vi "WriteStoreDataIngoHeucke.vi"(1 "Spots":T1[](array[typedef]) {"F2-Value overall" format="%.2f"; "tauerror" format="%.2f"; "Lifetime[ns]" format="%.2f"; "F2-Value TAC" format="%.2f"}, 2 "Enum":enum16{"Save", "Control"}(ring), 3 "Image Path":refnum<vi>) -> (0 "already x spots":i16)   [LabVIEW 2009]
uses:
  spotproperties.ctl
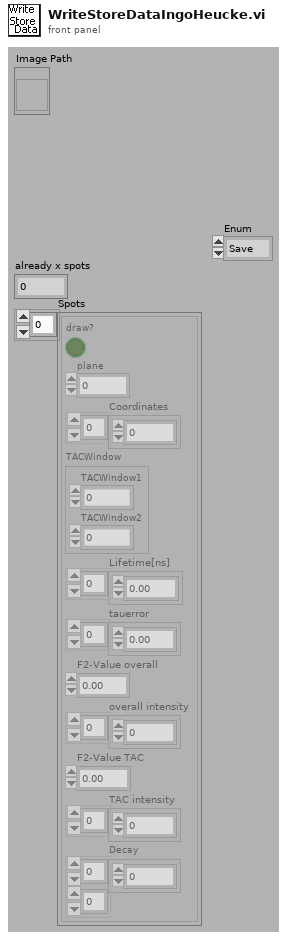
[diagram p1: front panel]
types:
  T1 = typedef "spotproperties.ctl" = cluster{"draw?":bool, "plane":u32, "Coordinates":i32[], "TACWindow":cluster{"TACWindow1":i32, "TACWindow2":i32}, "Lifetime[ns]":ext[], "tauerror":dbl[], "F2-Value overall":dbl, "overall intensity":u32[], "F2-Value TAC":dbl, "TAC intensity":u32[], "Decay":u32[][]}
  T2 = enum16{"Display", "change", "Get", "Set", "Set Ken"}
  T3 = enum16{"open", "open or create", "create or replace", "create", "open (read only)"}
  T4 = enum16{"read/write", "read-only", "write-only", "write-only (truncate)"}
  T5 = typedef "Settings.ctl" = cluster{"threshold":cluster{"max":u32, "min":u32}, "RGB or false color":bool, "16bit":bool, "log/lin axis":u16, "spotsize button":bool, "Pixelsize":u16, "autoscale x":bool, "autoscale y":bool, "correlation":bool, "ADC-Resolution":i32, "F2-lifetime":cluster{"display tau":bool, "display F2":bool, "Palette Number lifetime":enum32{"Gray", "Binary", "Gradient", "Rainbow", "Temperature"}, "Palette Number F2":enum32{"Gray", "Binary", "Gradient", "Rainbow", "Temperature"}, "max tau-Value":dbl, "min tau-Value":dbl, "max F2-Value":dbl, "min F2-Value":dbl}, "TAC-Window 1":u16, "TAC-Window 2":u16, "false color palette":cluster{"1":u32, "2":u32, "3":u32, "4":u32, "5":u32, "6":u32, "7":u32, "8":u32, "8 2":u32, "8 3":u32, "8 4":u32, "8 5":u32}}
  T6 = typedef "FIFOSettings_BH.ctt" = cluster{"Measurement":cluster{"Binning (ms)":sgl, "External Trigger Condition":u16, "Stop Condition:":u16, "Stop Count":dbl, "Buffer Size (Photons)":u16, "No of Channels":u16, "Ext Latch Delay":i16}, "ADC":cluster{"Module":u16, "ADC Resolution":i32, "Dither Range":i16, "Count Increment":i16, "Macro Time Clock":i16}, "SYNC":cluster{"SYNC ZC Level (mV)":sgl, "SYNC Freq Divider":i16, "SYNC Holdoff (ns)":sgl, "SYNC Threshold (mV)":sgl}, "TAC":cluster{"TAC Range (ns)":sgl, "TAC Gain":i16, "TAC Offset (%)":sgl, "TAC Limit Low (%)":sgl, "TAC Limit High (%)":sgl}, "CFD":cluster{"CFD Limit Low (mV)":sgl, "CFD Limit High (mV)":sgl, "CFD ZC Level (mV)":sgl, "CFD Holdoff (ns)":sgl}}
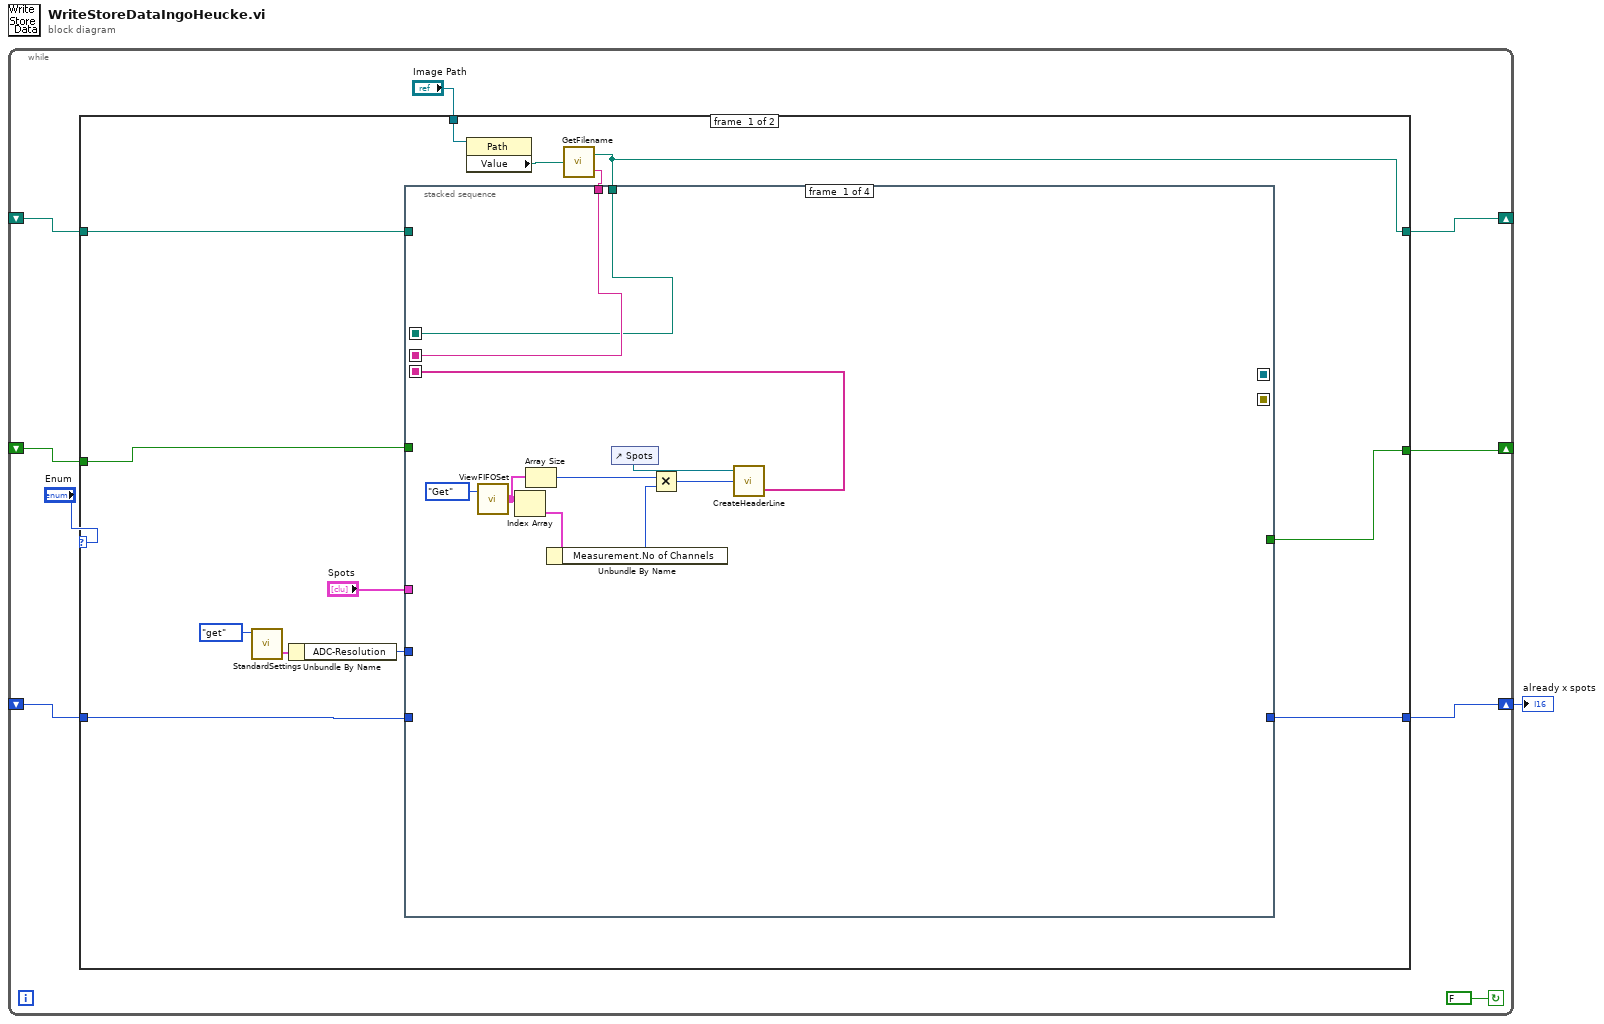
[diagram p0: block diagram]
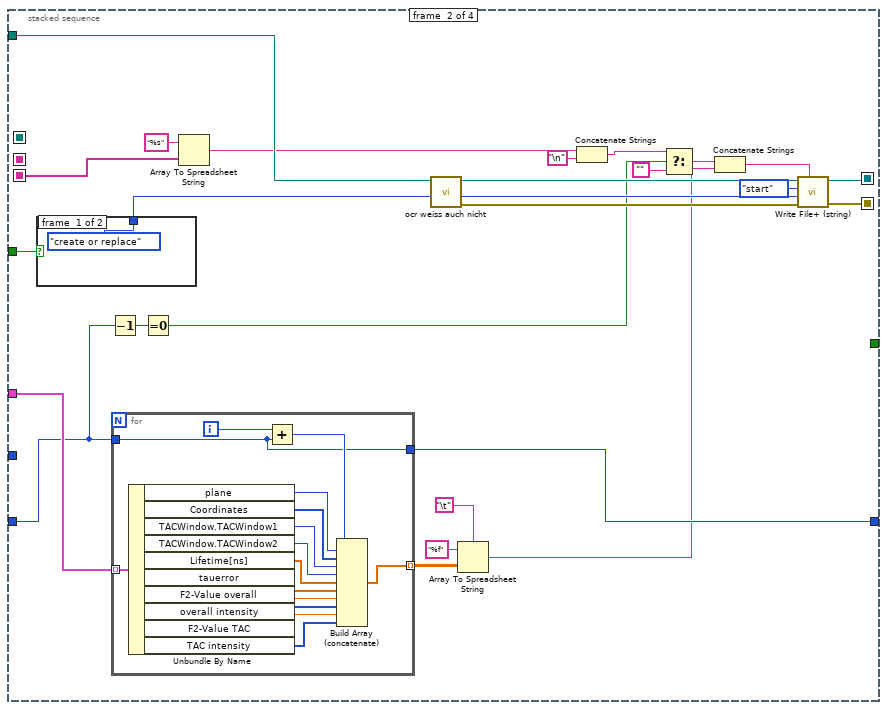
[diagram p2: hidden frame]
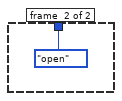
[diagram p3: hidden frame]
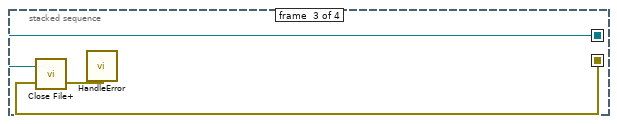
[diagram p4: hidden frame]
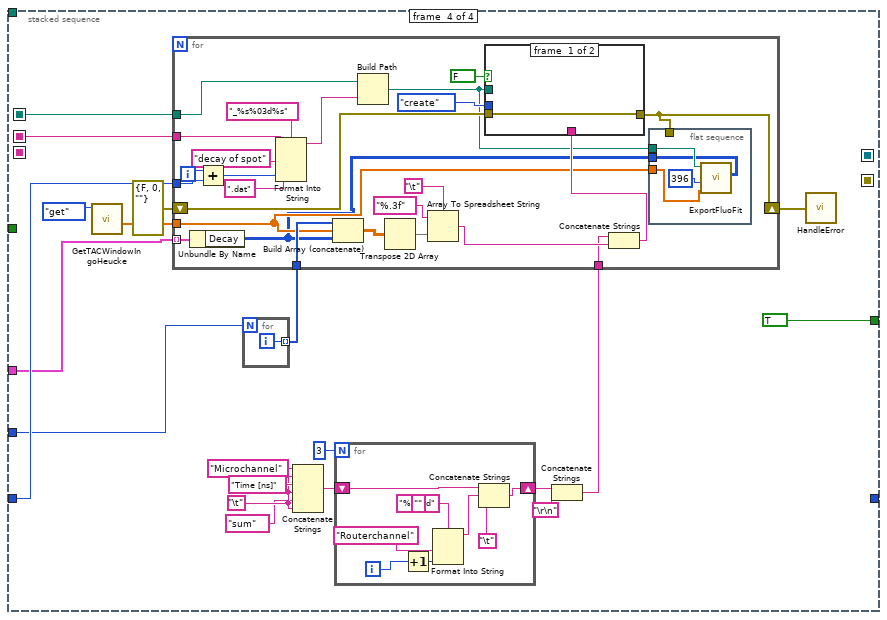
[diagram p5: hidden frame]
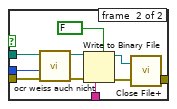
[diagram p6: hidden frame]
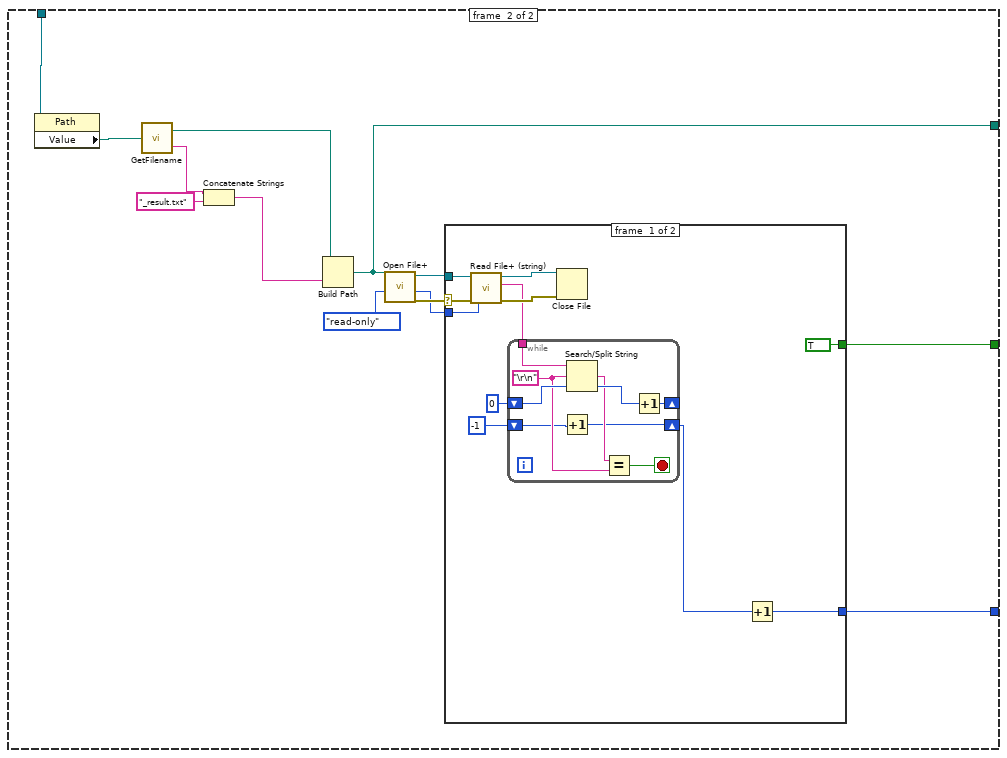
[diagram p7: hidden frame]
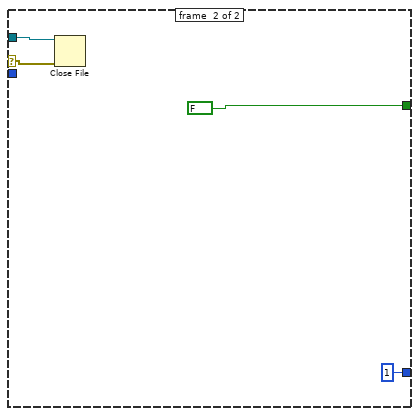
[diagram p8: hidden frame]
diagram:
  n1 = while {
    shift-right: [w8] -> _
    shift-left: _ -> [w7]
    shift-right: [w6] -> w1
    shift-left: _ -> [w5]
    shift-right: [w4] -> _
    shift-left: _ -> [w3]
    stop <- FALSE continue-if-true
    n2 = case shown="\"Save\", Default" "Enum" {
      tunnel: [w23 w161] -> w8
      tunnel: w7 -> [w22 _]
      tunnel: [w21 w149] -> w6
      tunnel: w5 -> [w15 _]
      tunnel: [w11 w151] -> w4
      tunnel: w3 -> [w20 _]
      tunnel: "Image Path" -> [w13 w150]
      frame #0 {
        n3 = call "StandardSettings.vi"("Enum"=enum16{"Load", "get", "Save", "set"}."get") -> ("StandardSettings"=w18:T5)  [unwired: 4 in]
        n4 = Unbundle By Name(w18) -> ("ADC-Resolution"=w17:i32)
        n5 = property class="Path"(reference=w13) -> ("Value"=w14:path)  [unwired: 1 in, 2 out]
        n6 = call "GetFilename.vi"("Value"=w14) -> ("base path"=w11:path, "name"=w12:string)
        n7 = stacked-sequence {
          seq-local: [w24 _ _ _] -> [_ _ _ w99]
          seq-local: [w25 _ _ _] -> [_ _ _ w87]
          seq-local: [w32 _ _ _] -> [_ w45 _ _]
          seq-local: [_ w58 _ _] -> [_ _ w79 _]
          seq-local: [_ w57 _ _] -> [_ _ w78 _]
          tunnel: "Spots" -> [_ w56 _ w84]
          tunnel: [_ _ _ TRUE] -> w23
          tunnel: w22 -> [_ w49 _ _]
          tunnel: [_ w48 _ _] -> w21
          tunnel: w15 -> [_ w41 _ w91]
          tunnel: w20 -> [_ w46 _ _]
          tunnel: w17 -> [_ _ _ w83]
          tunnel: w12 -> [w25 _ _ _]
          tunnel: w11 -> [w24 _ _ _]
          frame #0 {
            n8 = call "ViewFIFOSet.vi"("Enum"=T2."Get") -> ("FIFO Settings (Array)"=w27:T6[])  [unwired: 1 in]
            n9 = Index Array(array=w27) -> (element=w30:T6)  [unwired: 1 in]
            n10 = Array Size(array=w27) -> (size(s)=w28:i32)
            n11 = Unbundle By Name(w30) -> ("Measurement.No of Channels"=w29:u16)
            n12 = control-ref of="Spots"() -> (w33:refnum<vi>)
            n13 = Multiply(x=w28, y=w29) -> (x*y=w26:i32)
            n14 = call "CreateHeaderLine.vi"("No of channels"=w26, "Spots 3"=w33) -> ("Headline array"=w32:string[])  [unwired: 2 in]
          }
          frame #1 {
            n15 = case shown="True" w49 {
              tunnel: [T3."create or replace" ("function (open:0)") T3."open" ("function (open:0)")] -> w59
              frame #0 {
              }
              frame #1 {
              }
            }
            n16 = Decrement(x=w41) -> (x-1=w42:i16)
            n17 = for {
              tunnel: w56 -> [w76] mode=indexing
              tunnel: [w75] -> w55 mode=indexing
              tunnel: [w72] -> w48
              tunnel: w41 -> [w72]
              i -> [w74]
              n18 = Unbundle By Name(w76) -> ("plane"=w71:u32, "Coordinates"=w70:i32[], "TACWindow.TACWindow1"=w69:i32, "TACWindow.TACWindow2"=w68:i32, "Lifetime[ns]"=w67:ext[], "tauerror"=w66:dbl[], "F2-Value overall"=w65:dbl, "overall intensity"=w64:u32[], "F2-Value TAC"=w63:dbl, "TAC intensity"=w62:u32[])
              n19 = Add(x=w74, y=w72) -> (x+y=w73:i32)
              n20 = Build Array (concatenate)(w73, w71, w70, w69, w68, w67, w66, w65, w64, w63, w62) -> (w75:ext[])
            }
            n21 = Equal To 0?(x=w42) -> (x = 0?=w40:bool)
            n22 = Array To Spreadsheet String(array=w45, 3:"%s" ("format string")) -> (spreadsheet string=w43:string)  [unwired: 1 in]
            n23 = call "ocr weiss auch nicht.vi"("function (open:0)"=w59, "file path"=w46) -> ("error out"=w52:errorcluster, "file size (bytes)"=w50:i32, "refnum"=w53:refnum<file>)  [unwired: 6 in, 1 out]
            n24 = Array To Spreadsheet String(delimiter (Tab)="\t", array=w55, 3:"%f" ("format string")) -> (spreadsheet string=w36:string)
            n25 = Concatenate Strings(w43, "\n") -> (w39:string)
            n26 = Select(t=w39, s=w40, f="") -> (s? t:f=w37:string)
            n27 = Concatenate Strings(w37, w36) -> (w35:string)
            n28 = call "Write File+ (string).vi"("string"=w35, "error in (no error)"=w52, "pos offset (bytes:0)"=w50, "pos mode (rel. to end:1)"=enum16{"start", "end", "current"}."start", "refnum"=w53) -> ("error out"=w57:errorcluster, "dup refnum"=w58:refnum<file>)  [unwired: 2 in, 1 out]
          }
          frame #2 {
            n29 = call "Close File+.vi"("error in (no error)"=w78, "refnum"=w79) -> ("error out"=w77:errorcluster)  [unwired: 3 in, 2 out]
            n30 = call "HandleError.vi"("error in (no error)"=w77) -> ()
          }
          frame #3 {
            w86 = "\t"
            n31 = call "GetTACWindowIngoHeucke.vi"("Enum"=enum16{"ini", "get", "quick"}."get") -> ("x-values"=w80:dbl[])  [unwired: 1 in, 8 out]
            n32 = for {
              N: w83 -> [_]
              tunnel: [w100] -> w89 mode=indexing
              i -> [w100]
            }
            n33 = Concatenate Strings("Microchannel" ("string"), w86, "Time [ns]" ("string"), w86, "sum" ("string"), w86) -> (w93:string)
            n34 = for {
              N: 3 -> [_]
              shift-right: [w108] -> w97
              shift-left: w93 -> [w107]
              i -> [w105]
              (unwired) "%s %d" ("format string")
              n35 = Increment(x=w105) -> (x+1=w104:i32)
              n36 = Format Into String(format string="", "Routerchannel", w104) -> (resulting string=w102:string)  [unwired: 2 in, 1 out]
              n37 = Concatenate Strings(w107, w102, "\t") -> (w108:string)
            }
            n38 = Concatenate Strings(w97, "\r\n") -> (w96:string)
            n39 = for {
              tunnel: w84 -> [w133] mode=indexing
              tunnel: w99 -> [w132]
              tunnel: w80 -> [w113]
              shift-right: [w111] -> w81
              shift-left: errorcluster {"status"=FALSE, "code"=0, "source"=""} ("error out") -> [w127]
              tunnel: w96 -> [w124]
              tunnel: w91 -> [w119]
              tunnel: w87 -> [w114]
              tunnel: w89 -> [w115]
              i -> [w120]
              n40 = Unbundle By Name(w133) -> ("Decay"=w109:u32[][])
              n41 = Add(x=w120, y=w119) -> (x+y=w118:i32)
              n42 = Format Into String(format string="_%s%03d%s", initial string=w114, "decay of spot", w118, ".dat" ("replace string (\"\")")) -> (resulting string=w122:string)  [unwired: 1 in, 1 out]
              n43 = Build Array (concatenate)(w115, w113, w109) -> (w130:dbl[][])
              n44 = Build Path(base path=w132, name or relative path=w122) -> (appended path=w112:path)
              n45 = Transpose 2D Array(2D array=w130) -> (transposed array=w129:dbl[][])
              n46 = Array To Spreadsheet String(delimiter (Tab)="\t", array=w129, 3:"%.3f" ("format string")) -> (spreadsheet string=w126:string)
              n47 = Concatenate Strings(w124, w126) -> (w125:string)
              n48 = case shown="False" FALSE {
                tunnel: w127 -> [w134 w140]
                tunnel: w125 -> [_ w139]
                tunnel: T3."create" ("function (open:0)") -> [_ w138]
                tunnel: w112 -> [_ w137]
                tunnel: [w134 w136] -> w111
                frame #0 {
                }
                frame #1 {
                  n49 = call "ocr weiss auch nicht.vi"("error in (no error)"=w140, "function (open:0)"=w138, "file path"=w137) -> ("error out"=w141:errorcluster, "refnum"=w142:refnum<file>)  [unwired: 5 in, 2 out]
                  n50 = Write to Binary File(file (use dialog)=w142, data=w139, error in=w141, 5:FALSE ("prepend array or string size? (T)")) -> (refnum out=w143:refnum<file>, error out=w144:errorcluster)  [unwired: 2 in, 1 out]
                  n51 = call "Close File+.vi"("error in (no error)"=w144, "refnum"=w143) -> ("error out"=w136:errorcluster)  [unwired: 3 in, 2 out]
                }
              }
              n52 = flat-sequence {
                tunnel: w113 -> [w148]
                tunnel: w112 -> [w147]
                tunnel: w111 -> [_]
                tunnel: w109 -> [w146]
                frame #0 {
                  n53 = call "ExportFluoFit.vi"("time in"=w148, "# of lines"=396, "lifetimes"=w146, "Lifetime Export Path (ASCII-File)"=w147) -> ()  [unwired: 1 in]
                }
              }
            }
            n54 = call "HandleError.vi"("error in (no error)"=w81) -> ()
          }
        }
      }
      frame #1 {
        n55 = property class="Path"(reference=w150) -> ("Value"=w156:path)  [unwired: 1 in, 2 out]
        n56 = call "GetFilename.vi"("Value"=w156) -> ("base path"=w154:path, "name"=w155:string)
        n57 = Concatenate Strings(w155, "_result.txt" ("string")) -> (w152:string)
        n58 = Build Path(base path=w154, name or relative path=w152) -> (appended path=w151:path)
        n59 = call "Open File+.vi"("open mode (read-only:1)"=T4."read-only", "file path (\" \")"=w151) -> ("error out"=w158:errorcluster, "file size (bytes)"=w157:i32, "refnum"=w159:refnum<file>)  [unwired: 6 in, 1 out]
        n60 = case shown="No Error" w158 {
          selector: w158 -> [w170 w182]
          tunnel: w159 -> [w171 w183]
          tunnel: [TRUE FALSE] -> w161
          tunnel: [w162 i16 1] -> w149
          tunnel: w157 -> [w164 _]
          frame #0 {
            n61 = call "Read File+ (string).vi"("count"=w164, "error in (no error)"=w170, "refnum"=w171) -> ("error out"=w168:errorcluster, "string"=w167:string, "dup refnum"=w169:refnum<file>)  [unwired: 4 in, 2 out]
            n62 = while {
              shift-right: [w173] -> _
              shift-left: 0 ("offset of match") -> [w179]
              shift-right: [w174] -> w163
              shift-left: i16 -1 -> [w175]
              tunnel: w167 -> [w181]
              stop <- w176 stop-if-true
              w177 = "\r\n"
              n63 = Increment(x=w175) -> (x+1=w174:i16)
              n64 = Search/Split String(string=w181, search string/char (-)=w177, offset (0)=w179) -> (match + rest of string=w178:string, offset of match=w180:i32)  [unwired: 1 out]
              n65 = Equal?(x=w178, y=w177) -> (x = y?=w176:bool)
              n66 = Increment(x=w180) -> (x+1=w173:i32)
            }
            n67 = Close File(refnum=w169, error in=w168) -> ()  [unwired: 2 out]
            n68 = Increment(x=w163) -> (x+1=w162:i16)
          }
          frame #1 {
            n69 = Close File(refnum=w183, error in=w182) -> ()  [unwired: 2 out]
          }
        }
      }
    }
  }
  "already x spots" <- w1
